vi "EEG_2022_040_LabView_1.1.vi"() -> ()   [LabVIEW 2022 SP3]
panel:
  out "Message":string
  out "Warning":bool
  out "Seconds":dbl
  out "Minutes":dbl
  out "Hours":dbl
  in  "Total Time in Seconds":dbl
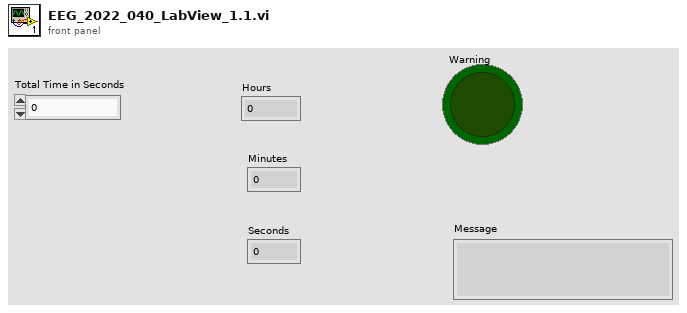
[diagram p1: front panel]
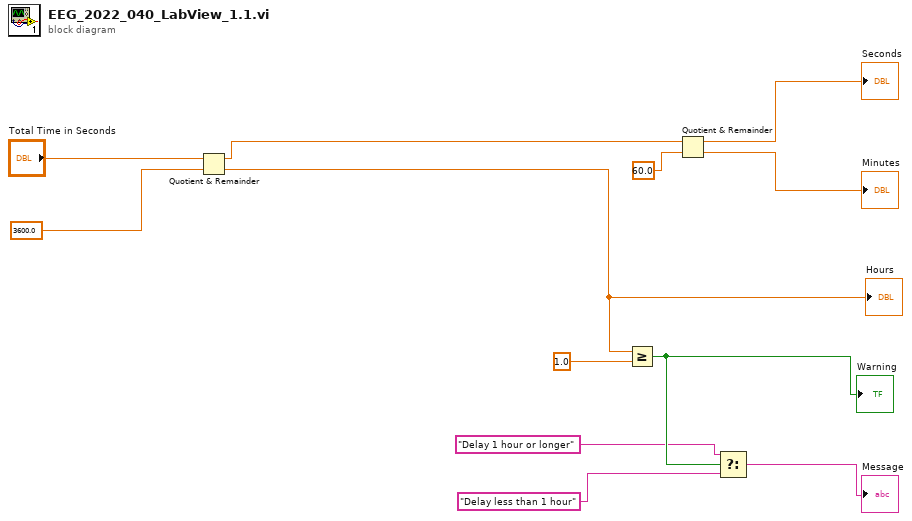
[diagram p0: block diagram]
diagram:
  n1 = Quotient & Remainder(x="Total Time in Seconds", y=3600.0) -> (x-y*floor(x/y)=w10:dbl, floor(x/y)=w7:dbl)
  "Hours" <- w7
  n2 = Greater Or Equal?(x=w7, y=1.0) -> (x >= y?=w5:bool)
  "Warning" <- w5
  n3 = Quotient & Remainder(x=w10, y=60.0) -> (x-y*floor(x/y)=→"Seconds":dbl, floor(x/y)=→"Minutes":dbl)
  n4 = Select(t="Delay 1 hour or longer", s=w5, f="Delay less than 1 hour") -> (s? t:f=→"Message":string)
